vi "Send Log Configuration.vi"(6 "log thresholds":T1 {"Segment Files By" items=["Time", "Size"]}, 7 "Timestamp":bool, 8 "error in":errorcluster, 9 "Base name":string, 10 "Log File Directory":string, 11 "Log Producer in":T2) -> (0 "error out":errorcluster, 3 "Log Producer out":T2)   [LabVIEW 2020, in "Frame Logging.lvlib"]
uses:
  Frame Logging.lvlib
  Log_Producer.ctl
  Message_Request.ctl
  Message_Request_Action.ctl
  Shared/loggingThreshold_types.ctl
  Log_Configuration.ctl
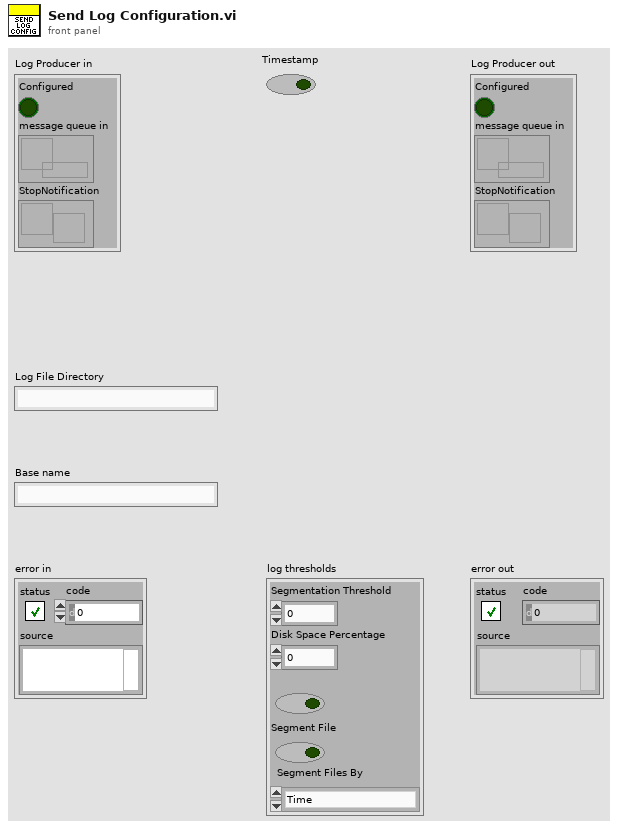
[diagram p1: front panel]
types:
  T1 = typedef "loggingThreshold_types.ctl" = cluster{"Segmentation Threshold":dbl, "Disk Space Percentage":dbl, "Check Disk Space":bool, "Segment File":bool, "Segment Files By":u16}
  T2 = typedef "Frame Logging.lvlib/Log_Producer.ctl" = cluster{"Configured":bool, "message queue in":refnum<queue>, "StopNotification":refnum<notifier>}
  T3 = typedef "Frame Logging.lvlib/Log_Configuration.ctl" = cluster{"Log File Directory":string, "Base name":string, "Timestamp":bool, "log thresholds":T1}
  T4 = typedef "Frame Logging.lvlib/Message_Request_Action.ctl" = enum16{"Initialize", "Open File", "Log", "Manage Disk", "Stop", "Close File", "Update Configuration"}
  T5 = typedef "Frame Logging.lvlib/Message_Request.ctl" = cluster{"request":T4, "data":variant}
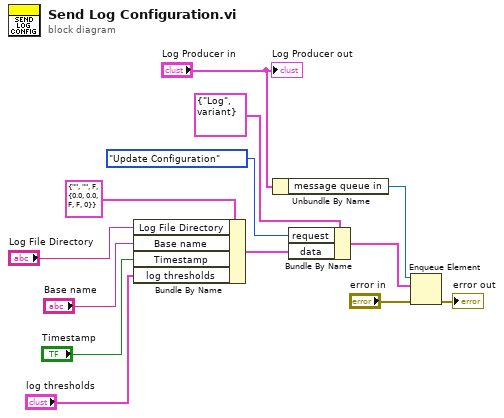
[diagram p0: block diagram]
diagram:
  n1 = Bundle By Name(cluster=T3 {"Log File Directory"="", "Base name"="", "Timestamp"=FALSE, "log thresholds"={"Segmentation Threshold"=0.0, "Disk Space Percentage"=0.0, "Check Disk Space"=FALSE, "Segment File"=FALSE, "Segment Files By"=0}} ("log configuration"), "Log File Directory"="Log File Directory", "Base name"="Base name", "Timestamp"="Timestamp", "log thresholds"="log thresholds") -> (w5:T3)
  n2 = Unbundle By Name("Log Producer in") -> ("message queue in"=w12:refnum<queue>)
  n3 = Bundle By Name(cluster=T5 {"request"=enum."Log", "data"=variant} ("Message_type"), "request"=Message_Request_Action."Update Configuration", "data"=w5) -> (w11:T5)
  n4 = Enqueue Element(queue=w12, element=w11, error in (no error)="error in") -> (error out=→"error out":errorcluster)  [unwired: 1 in, 2 out]
  "Log Producer out" <- "Log Producer in"
